vi "原始值工程转换.vi"(10 "工程量转换":T2={"原始值最小值"=0.0, "原始值最大值"=1.0, "转换值最小值"=0.0, "转换值最大值"=1.0, "原始值最小值 2"=0.0, "原始值最大值 2"=1.0, "转换值最小值 2"=0.0, "转换值最大值 2"=1.0, "原始值最小值 3"=0.0, "原始值最大值 3"=1.0, "转换值最小值 3"=0.0, "转换值最大值 3"=1.0, "原始值最小值 4"=0.0, "原始值最大值 4"=1.0, "转换值最小值 4"=0.0, "转换值最大值 4"=1.0, "原始值最小值 5"=0.0, "原始值最大值 5"=1.0, "转换值最小值 5"=0.0, "转换值最大值 5"=1.0, "原始值最小值 6"=0.0, "原始值最大值 6"=1.0, "转换值最小值 6"=0.0, "转换值最大值 6"=1.0, "原始值最小值 7"=0.0, "原始值最大值 7"=1.0, "转换值最小值 7"=0.0, "转换值最大值 7"=1.0, "原始值最小值 8"=0.0, "原始值最大值 8"=1.0, "转换值最小值 8"=0.0, "转换值最大值 8"=1.0} {"转换值最大值 8" format="%#.2f"; "转换值最小值 8" format="%#.2f"; "原始值最大值 8" format="%#.2f"; "原始值最小值 8" format="%#.2f"; "转换值最大值 7" format="%#.2f"; "转换值最小值 7" format="%#.2f"; "原始值最大值 7" format="%#.2f"; "原始值最小值 7" format="%#.2f"; "转换值最大值 6" format="%#.2f"; "转换值最小值 6" format="%#.2f"; "原始值最大值 6" format="%#.2f"; "原始值最小值 6" format="%#.2f"; "转换值最大值 5" format="%#.2f"; "转换值最小值 5" format="%#.2f"; "原始值最大值 5" format="%#.2f"; "原始值最小值 5" format="%#.2f"; "转换值最大值 4" format="%#.2f"; "转换值最小值 4" format="%#.2f"; "原始值最大值 4" format="%#.2f"; "原始值最小值 4" format="%#.2f"; "转换值最大值 3" format="%#.2f"; "转换值最小值 3" format="%#.2f"; "原始值最大值 3" format="%#.2f"; "原始值最小值 3" format="%#.2f"; "转换值最大值 2" format="%#.2f"; "转换值最小值 2" format="%#.2f"; "原始值最大值 2" format="%#.2f"; "原始值最小值 2" format="%#.2f"; "转换值最大值" format="%#.2f"; "转换值最小值" format="%#.2f"; "原始值最大值" format="%#.2f"; "原始值最小值" format="%#.2f"}, 11 "AD当前原始值":T1 {"AD7" format="%.2f"; "AD6" format="%.2f"; "AD5" format="%.2f"; "AD4" format="%.2f"; "AD3" format="%.2f"; "AD2" format="%.2f"; "AD1" format="%.2f"; "AD0" format="%.2f"}) -> (3 "AD当前转换值":T1 {"AD7" format="%.2f"; "AD6" format="%.2f"; "AD5" format="%.2f"; "AD4" format="%.2f"; "AD3" format="%.2f"; "AD2" format="%.2f"; "AD1" format="%.2f"; "AD0" format="%.2f"})   [LabVIEW 2016, in "环境动力单元.lvlib"]
panel:
  # "原始低值"
  # "原始高值"
  # "转换低值"
  # "转换高值"
  # "AD7:"
  # "AD6:"
  # "AD5:"
  # "AD4:"
  # "AD3:"
  # "AD2:"
  # "AD1:"
  # "AD0:"
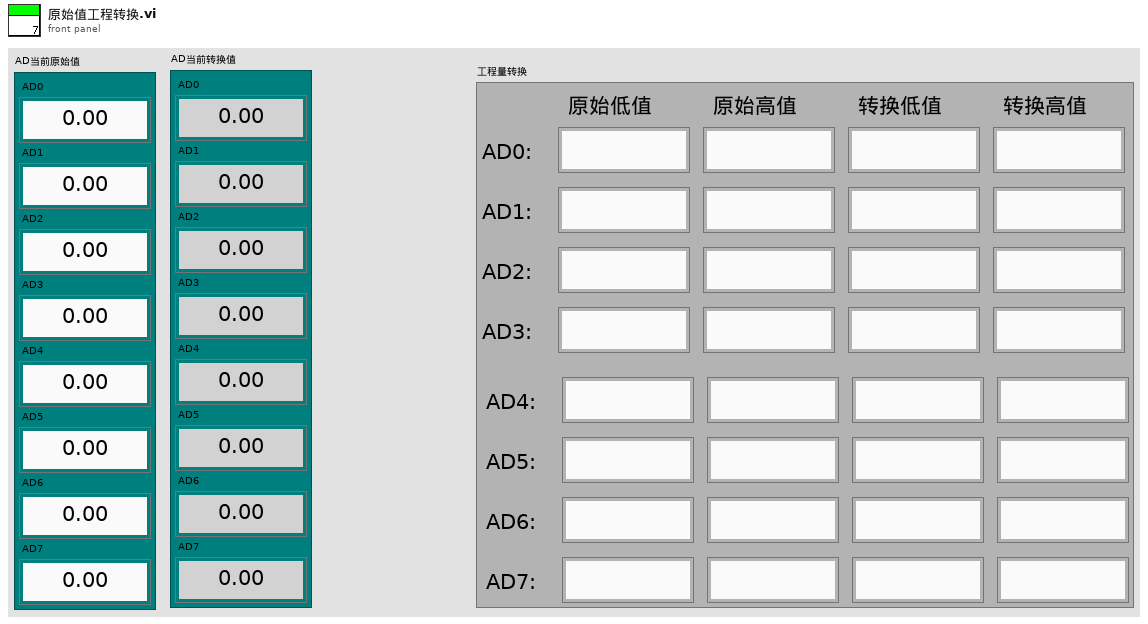
[diagram p1: front panel]
types:
  T1 = cluster{"AD0":dbl, "AD1":dbl, "AD2":dbl, "AD3":dbl, "AD4":dbl, "AD5":dbl, "AD6":dbl, "AD7":dbl}
  T2 = cluster{"原始值最小值":dbl, "原始值最大值":dbl, "转换值最小值":dbl, "转换值最大值":dbl, "原始值最小值 2":dbl, "原始值最大值 2":dbl, "转换值最小值 2":dbl, "转换值最大值 2":dbl, "原始值最小值 3":dbl, "原始值最大值 3":dbl, "转换值最小值 3":dbl, "转换值最大值 3":dbl, "原始值最小值 4":dbl, "原始值最大值 4":dbl, "转换值最小值 4":dbl, "转换值最大值 4":dbl, "原始值最小值 5":dbl, "原始值最大值 5":dbl, "转换值最小值 5":dbl, "转换值最大值 5":dbl, "原始值最小值 6":dbl, "原始值最大值 6":dbl, "转换值最小值 6":dbl, "转换值最大值 6":dbl, "原始值最小值 7":dbl, "原始值最大值 7":dbl, "转换值最小值 7":dbl, "转换值最大值 7":dbl, "原始值最小值 8":dbl, "原始值最大值 8":dbl, "转换值最小值 8":dbl, "转换值最大值 8":dbl}
  T3 = cluster{"数组[0]":dbl, "数组[1]":dbl, "数组[2]":dbl, "数组[3]":dbl, "数组[4]":dbl, "数组[5]":dbl, "数组[6]":dbl, "数组[7]":dbl}
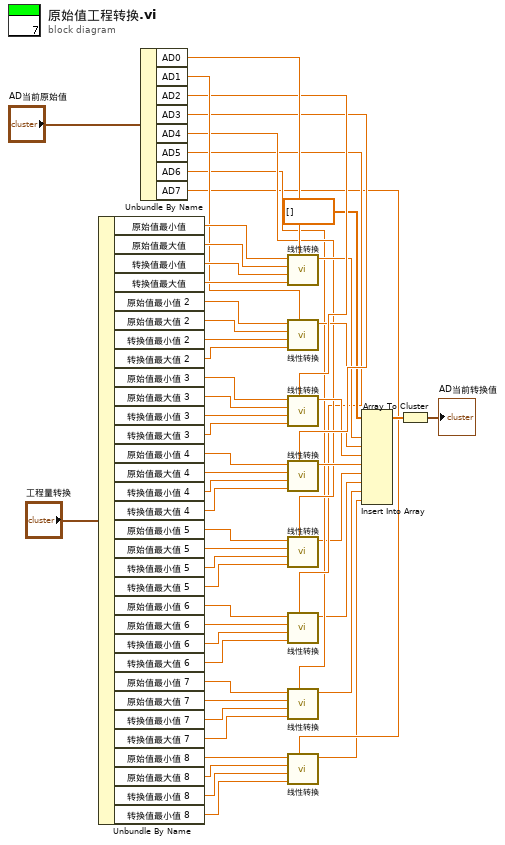
[diagram p0: block diagram]
diagram:
  n1 = Unbundle By Name("工程量转换") -> ("原始值最小值"=w51:dbl, "原始值最大值"=w50:dbl, "转换值最小值"=w49:dbl, "转换值最大值"=w48:dbl, "原始值最小值 2"=w36:dbl, "原始值最大值 2"=w37:dbl, "转换值最小值 2"=w38:dbl, "转换值最大值 2"=w39:dbl, "原始值最小值 3"=w40:dbl, "原始值最大值 3"=w41:dbl, "转换值最小值 3"=w42:dbl, "转换值最大值 3"=w43:dbl, "原始值最小值 4"=w47:dbl, "原始值最大值 4"=w46:dbl, "转换值最小值 4"=w45:dbl, "转换值最大值 4"=w44:dbl, "原始值最小值 5"=w9:dbl, "原始值最大值 5"=w10:dbl, "转换值最小值 5"=w11:dbl, "转换值最大值 5"=w12:dbl, "原始值最小值 6"=w13:dbl, "原始值最大值 6"=w14:dbl, "转换值最小值 6"=w15:dbl, "转换值最大值 6"=w16:dbl, "原始值最小值 7"=w17:dbl, "原始值最大值 7"=w18:dbl, "转换值最小值 7"=w19:dbl, "转换值最大值 7"=w20:dbl, "原始值最小值 8"=w21:dbl, "原始值最大值 8"=w22:dbl, "转换值最小值 8"=w23:dbl, "转换值最小值 8"=w24:dbl)
  n2 = Unbundle By Name("AD当前原始值") -> ("AD0"=w35:dbl, "AD1"=w34:dbl, "AD2"=w33:dbl, "AD3"=w32:dbl, "AD4"=w8:dbl, "AD5"=w7:dbl, "AD6"=w6:dbl, "AD7"=w5:dbl)
  n3 = call "线性转换.vi"("AD0"=w35, "转换值最大值"=w48, "转换值最小值"=w49, "原始值最大值"=w50, "原始值最小值"=w51) -> ("数值"=w31:dbl)  [unwired: 6 in]
  n4 = call "线性转换.vi"("AD0"=w34, "转换值最大值"=w39, "转换值最小值"=w38, "原始值最大值"=w37, "原始值最小值"=w36) -> ("数值"=w29:dbl)  [unwired: 6 in]
  n5 = call "线性转换.vi"("AD0"=w33, "转换值最大值"=w43, "转换值最小值"=w42, "原始值最大值"=w41, "原始值最小值"=w40) -> ("数值"=w28:dbl)  [unwired: 6 in]
  n6 = call "线性转换.vi"("AD0"=w32, "转换值最大值"=w44, "转换值最小值"=w45, "原始值最大值"=w46, "原始值最小值"=w47) -> ("数值"=w27:dbl)  [unwired: 6 in]
  n7 = call "线性转换.vi"("AD0"=w8, "转换值最大值"=w12, "转换值最小值"=w11, "原始值最大值"=w10, "原始值最小值"=w9) -> ("数值"=w4:dbl)  [unwired: 6 in]
  n8 = call "线性转换.vi"("AD0"=w7, "转换值最大值"=w16, "转换值最小值"=w15, "原始值最大值"=w14, "原始值最小值"=w13) -> ("数值"=w3:dbl)  [unwired: 6 in]
  n9 = call "线性转换.vi"("AD0"=w6, "转换值最大值"=w20, "转换值最小值"=w19, "原始值最大值"=w18, "原始值最小值"=w17) -> ("数值"=w2:dbl)  [unwired: 6 in]
  n10 = call "线性转换.vi"("AD0"=w5, "转换值最大值"=w24, "转换值最小值"=w23, "原始值最大值"=w22, "原始值最小值"=w21) -> ("数值"=w1:dbl)  [unwired: 6 in]
  n11 = Insert Into Array(array=dbl[] [] ("数组"), new element #1=w31, new element #2=w29, new element #3=w28, new element #4=w27, new element #5=w4, new element #6=w3, new element #7=w2, new element #8=w1) -> (w26:dbl[])  [unwired: 1 in]
  n12 = Array To Cluster(array=w26) -> (cluster=→"AD当前转换值":T3)
